vi "test_Connector Pane.vi"(8 "error in (no error)":errorcluster, 11 "TestCase in":refnum<class "FPGA Addon Generic Tests.lvclass">) -> (0 "error out":errorcluster, 3 "TestCase out":refnum<class "FPGA Addon Generic Tests.lvclass">)   [LabVIEW 2019, in "FPGA Addon Generic Tests.lvclass"]
uses:
  FPGA Addon Generic Tests.lvclass
  <vilib>/addons/_JKI Toolkits/VI Tester/TestCase.llb/TestCase.lvclass
  C:/Program Files (x86)/National Instruments/LabVIEW 2019/vi.lib/addons/_JKI Toolkits/VI Tester/TestCase.llb/TestCase.lvclass
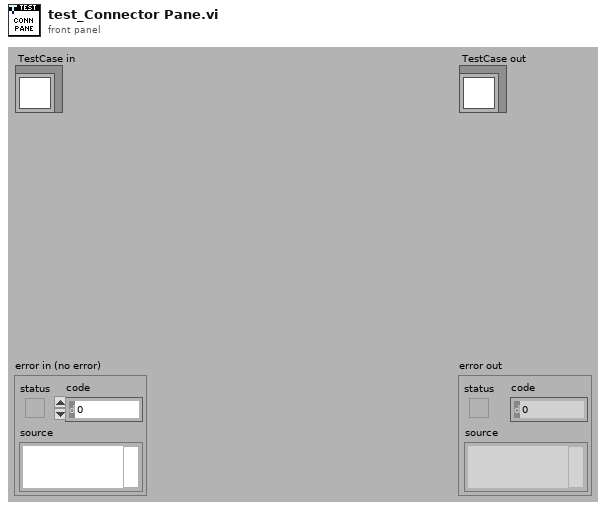
[diagram p1: front panel]
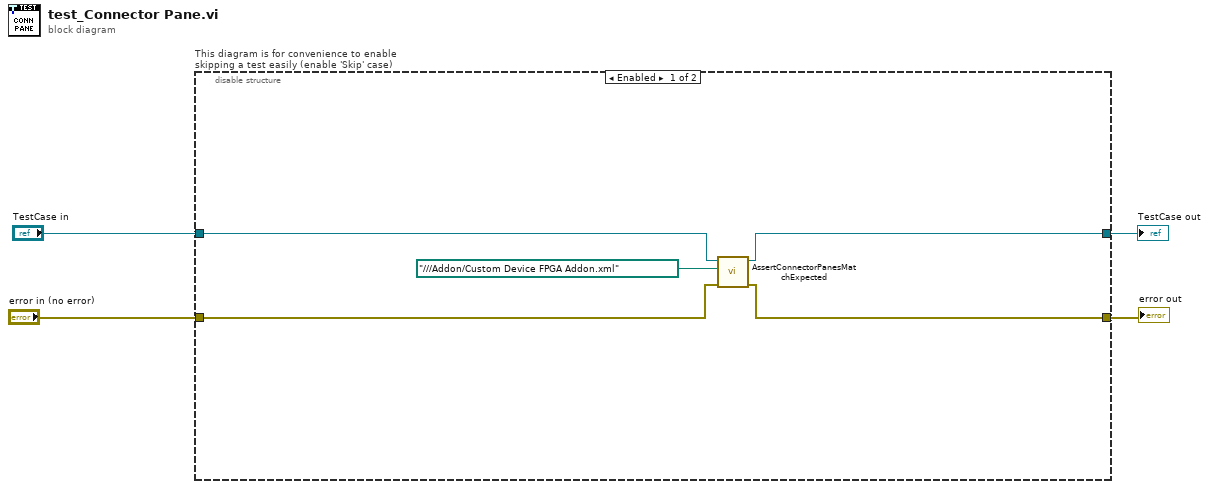
[diagram p0: block diagram]
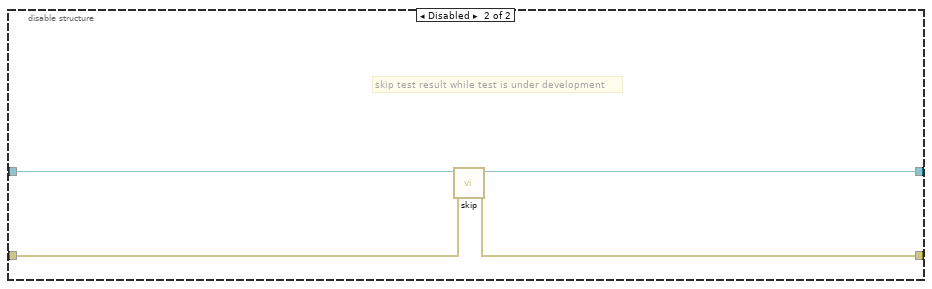
[diagram p2: hidden frame]
diagram:
  n1 = disable-structure "This diagram is for convenience to enable skipping a test easily (enable 'Skip' case)" shown="Enabled" {
    disable-tunnel: "TestCase in" -> [w9 w13]
    disable-tunnel: [w8 w11] -> w1
    disable-tunnel: [w6 w12] -> w3
    disable-tunnel: "error in (no error)" -> [w7 w10]
    frame Enabled {
      n2 = call "AssertConnectorPanesMatchExpected.vi"("error in (no error)"=w7, "custom device xml path"=path "../../../Addon/Custom Device FPGA Addon.xml" ("search path"), "TestCase in"=w9) -> ("error out"=w6:errorcluster, "TestCase out"=w8:refnum<class "FPGA Addon Generic Tests.lvclass">)  [unwired: 7 in]
    }
    frame Disabled {
      # "skip test result while test is under development"
      n3 = call <vilib>:"skip.vi"("error in (no error)"=w10, "TestCase in"=w13) -> ("error out"=w12:errorcluster, "TestCase out"=w11:refnum<class "FPGA Addon Generic Tests.lvclass">)  [unwired: 8 in]
    }
  }
  "error out" <- w3
  "TestCase out" <- w1
